vi "Hide_Channel_value.vi"(1 "Hide Values":bool, 2 "Hide if this Value":dbl=1.234e-06 format="%.9f", 3 "Value In":dbl format="%.2f") -> (0 "Value Out":dbl format="%.2f")   [LabVIEW 2010]
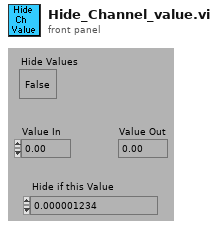
[diagram p1: front panel]
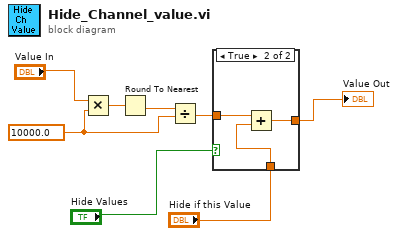
[diagram p0: block diagram]
diagram:
  w4 = 10000.0 ("y")
  n1 = Multiply(x="Value In", y=w4) -> (x*y=w6:dbl)
  n2 = Round To Nearest(number=w6) -> (nearest integer value=w5:dbl)
  n3 = Divide(x=w5, y=w4) -> (x/y=w3:dbl)
  n4 = case shown="True" "Hide Values" {
    tunnel: w3 -> [w9 w12]
    tunnel: "Hide if this Value" -> [_ w11]
    tunnel: [w9 w10] -> w2
    frame False {
    }
    frame True {
      n5 = Add(x=w12, y=w11) -> (x+y=w10:dbl)
    }
  }
  "Value Out" <- w2
